vi "NMEA断电保存全局变量.vi"() -> ()   [LabVIEW 2016, in "环境动力监测库.lvlib" / "NMEA.lvlib"]
uses:
  NMEA.lvlib
panel:
  in  "收方地址":string="968314"
  in  "GPS移位报警设定值":dbl=1000.0
  in  "BD移位报警设定值":dbl=1000.0
  in  "GPS波特率":u32(ring)=115200 items=["4800"=4800, "9600"=9600, "38400"=38400, "19200"=19200, "115200"=115200]
  in  "GPS VISA资源名称":refnum<visa-resource-name>
  in  "BD波特率":u32(ring)=115200 items=["4800"=4800, "9600"=9600, "38400"=38400, "19200"=19200, "115200"=115200]
  in  "BDVISA资源名称":refnum<visa-resource-name>
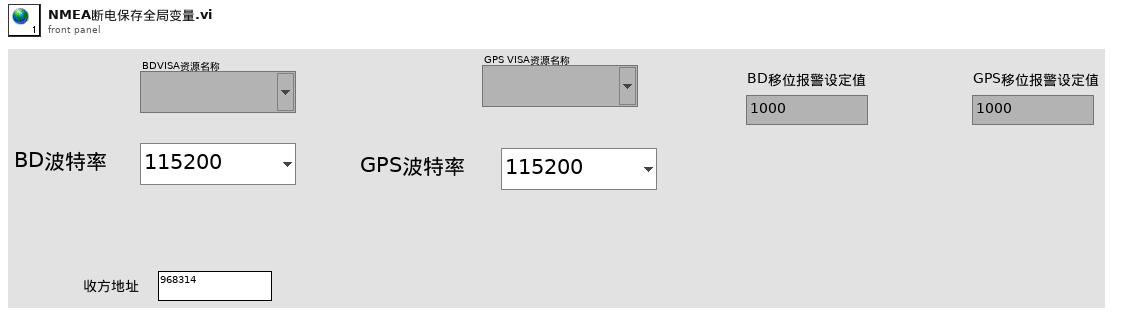
[diagram p1: front panel]
diagram:
